vi "Keithley 2002 Syst Commands.vi"(0 "GPIB address":string="16", 1 "Set Time &\nDate":bool, 2 "Reset\nRelative TimeStamp":bool, 3 "Reset\nReading Number":bool, 4 "TimeStamp Type":u16(ring) items=["Relative", "Real-Time Clock"], 5 "error in":T1, 6 "Reset":bool, 7 "Continue":bool=TRUE, 8 "Hours":string="12", 9 "Year":string="1994", 10 "Minutes":string="00", 11 "Month":string="08", 12 "Seconds":string="00", 13 "Day":string="01", 14 "line sync":bool, 15 "autozero (normal:0)":u16(ring) items=["normal", "synchronous", "disable"]) -> (19 "error out":T1)   [LabVIEW 2020]
doc: "This VI is used to perform some of the basic system commands. These commands are optional and do not need to be performed for any specified type of measurement."
panel:
  # "on\noff"
  # "on\noff"
  # "on\noff"
  # "on\noff"
  # "on\noff"
  # "enable\ndisable"
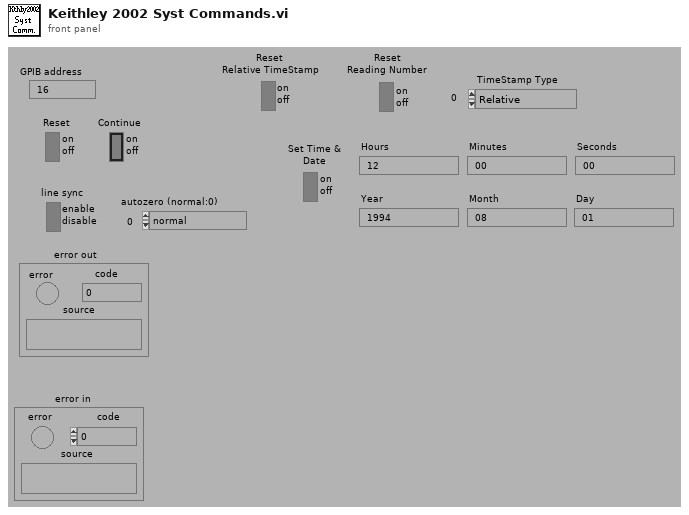
[diagram p1: front panel]
types:
  T1 = cluster{"error":bool, "code":i32, "source":string}
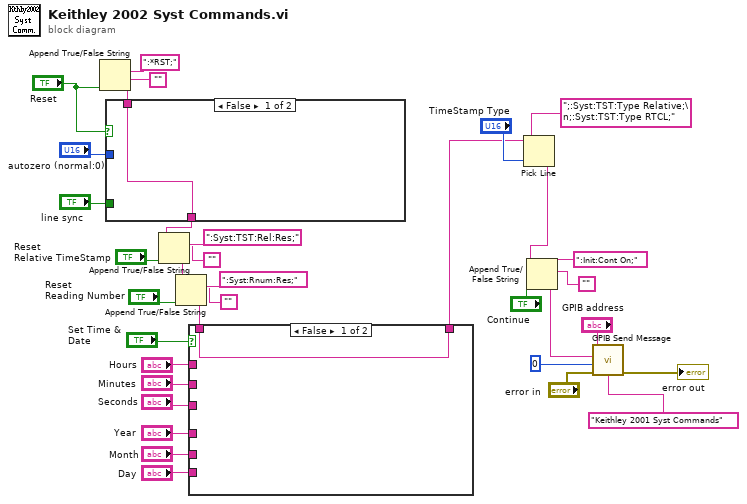
[diagram p0: block diagram]
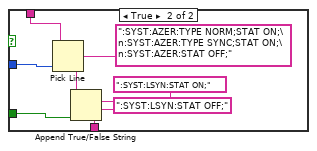
[diagram p2: hidden frame]
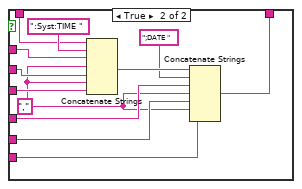
[diagram p3: hidden frame]
diagram:
  n1 = Append True/False String(1:"Reset", 2:"", 3:":*RST;") -> (0:w10:string)  [unwired: 1 in]
  n2 = case shown="False" "Reset" {
    tunnel: w10 -> [w36 w40]
    tunnel: [w36 w39] -> w9
    tunnel: "autozero (normal:0)" -> [_ w38]
    tunnel: "line sync" -> [_ w37]
    frame False {
    }
    frame True {
      n3 = Pick Line(string ("")=w40, multi-line string=":SYST:AZER:TYPE NORM;STAT ON;\n:SYST:AZER:TYPE SYNC;STAT ON;\n:SYST:AZER:STAT OFF;", line index=w38) -> (output string=w41:string)
      n4 = Append True/False String(1:w37, 2:":SYST:LSYN:STAT OFF;", 3:":SYST:LSYN:STAT ON;", 4:w41) -> (0:w39:string)
    }
  }
  n5 = Append True/False String(1:"Reset\nRelative TimeStamp", 2:"", 3:":Syst:TST:Rel:Res;", 4:w9) -> (0:w23:string)
  n6 = Append True/False String(1:"Reset\nReading Number", 2:"", 3:":Syst:Rnum:Res;", 4:w23) -> (0:w20:string)
  n7 = case shown="False" "Set Time &\nDate" {
    tunnel: w20 -> [w45 w54]
    tunnel: "Hours" -> [_ w53]
    tunnel: "Minutes" -> [_ w52]
    tunnel: "Seconds" -> [_ w51]
    tunnel: "Year" -> [_ w50]
    tunnel: "Month" -> [_ w49]
    tunnel: "Day" -> [_ w47]
    tunnel: [w45 w46] -> w2
    frame False {
    }
    frame True {
      w48 = ","
      n8 = Concatenate Strings(w54, ":Syst:TIME ", w53, w48, w52, w48, w51) -> (w56:string)
      n9 = Concatenate Strings(w56, ";DATE ", w50, w48, w49, w48, w47) -> (w46:string)
    }
  }
  n10 = Pick Line(string ("")=w2, multi-line string=";:Syst:TST:Type Relative;\n;:Syst:TST:Type RTCL;", line index="TimeStamp Type") -> (output string=w1:string)
  n11 = Append True/False String(1:"Continue", 2:"", 3:":Init:Cont On;", 4:w1) -> (0:w5:string)
  n12 = call "GPIB Send Message.vi"("address string"="GPIB address", "write buffer"=w5, "source"="Keithley 2001 Syst Commands", "write mode (set END:0)"=0, "error in"="error in") -> ("error out"=→"error out":T1)  [unwired: 2 in, 2 out]
